vi "ADCP过程数据.vi"(7 "电压":sgl, 8 "Error in":errorcluster caption="Error in (no error)", 9 "纵摇":sgl, 10 "横摇":sgl, 11 "时间":timestamp) -> (0 "错误输出":errorcluster)   [LabVIEW 2016, in "ADCP.lvlib"]
uses:
  ADCP.lvlib
panel:
  out "data":T1
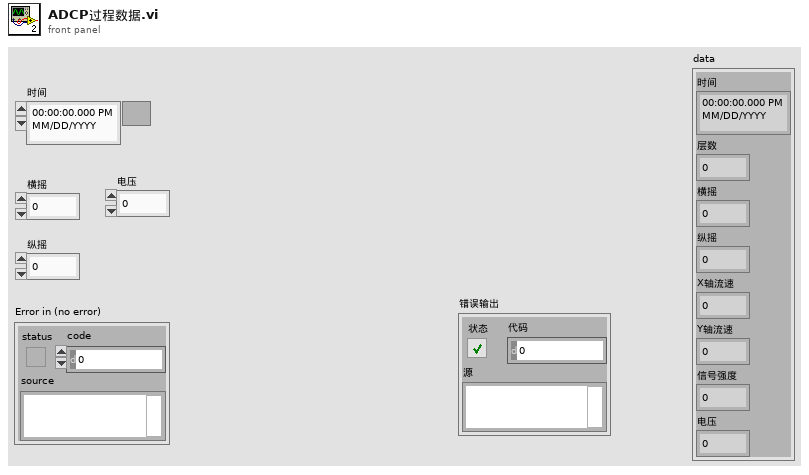
[diagram p1: front panel]
types:
  T1 = cluster{"时间":timestamp, "层数":u16, "横摇":sgl, "纵摇":sgl, "X轴流速":sgl, "Y轴流速":sgl, "信号强度":u16, "电压":sgl}
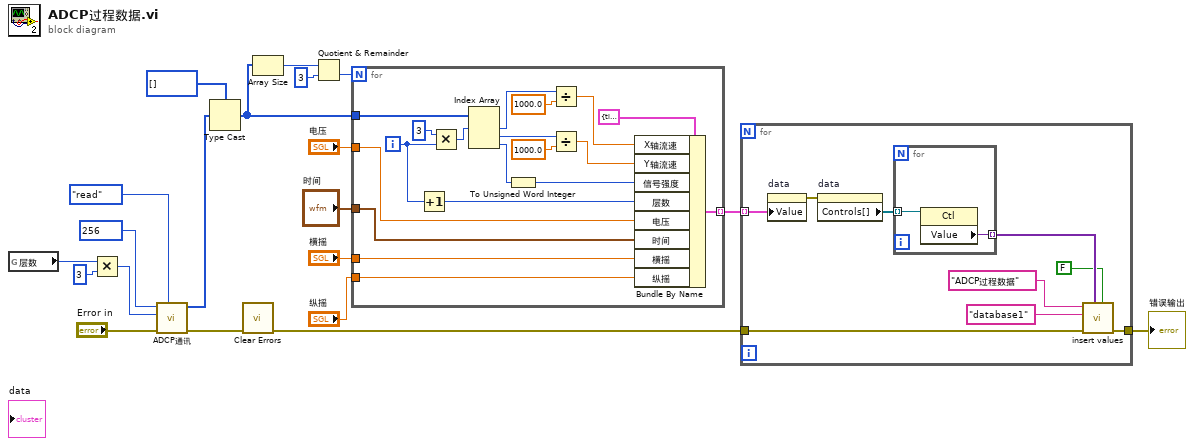
[diagram p0: block diagram]
diagram:
  n1 = global read "ADCP全局变量.vi" "层数"() -> (w19:u16)
  n2 = Multiply(x=w19, y=u16 3) -> (x*y=w17:u16)
  n3 = call "ADCP通讯.vi"("STEP"=enum16{"open", "read", "write", "close"}."read", "Error in"="Error in", "quantity"=w17, "starting address"=u16 256) -> ("error out"=w2:errorcluster, "Registers"=w10:u16[])  [unwired: 5 in, 1 out]
  n4 = Type Cast(type=i16[] [], x=w10) -> (*(type *) &x=w14:i16[])
  n5 = call <vilib>:"Clear Errors.vi"("error in (no error)"=w2) -> ("error out"=w1:errorcluster)  [unwired: 5 in, 1 out]
  n6 = Array Size(array=w14) -> (size(s)=w13:i32)
  n7 = Quotient & Remainder(x=w13, y=3) -> (floor(x/y)=w11:i32)  [unwired: 1 out]
  n8 = for {
    N: w11 -> [_]
    tunnel: w14 -> [w39]
    tunnel: [w27] -> w6 mode=indexing
    tunnel: "电压" -> [w26]
    tunnel: "时间" -> [w25]
    tunnel: "横摇" -> [w24]
    tunnel: "纵摇" -> [w23]
    i -> [w22]
    n9 = Increment(x=w22) -> (x+1=w21:i32)
    n10 = Multiply(x=3, y=w22) -> (x*y=w37:i32)
    n11 = Index Array(array=w39, index #1=w37) -> (element #1=w36:i16, element #2=w33:i16, element #3=w32:i16)  [unwired: 2 in]
    n12 = To Unsigned Word Integer(number=w32) -> (unsigned 16bit integer=w28:u16)
    n13 = Divide(x=w36, y=sgl 1000.0) -> (x/y=w30:sgl)
    n14 = Divide(x=w33, y=sgl 1000.0) -> (x/y=w29:sgl)
    n15 = Bundle By Name(cluster=T1 {"时间"=timestamp(0 s since 1904-01-01), "层数"=0, "横摇"=0.0, "纵摇"=0.0, "X轴流速"=0.0, "Y轴流速"=0.0, "信号强度"=0, "电压"=0.0}, "X轴流速"=w30, "Y轴流速"=w29, "信号强度"=w28, "层数"=w21, "电压"=w26, "时间"=w25, "横摇"=w24, "纵摇"=w23) -> (w27:T1)
  }
  n16 = for {
    tunnel: w6 -> [w46] mode=indexing
    tunnel: w1 -> [w41]
    tunnel: [w40] -> w4
    n17 = property on="data" class="Clust (严格)"("Value"=w46) -> (error out=w45:errorcluster)  [unwired: 2 in, 1 out]
    n18 = property on="data" class="Clust (严格)"(error in=w45) -> ("Controls[]"=w44:refnum<vi>[])  [unwired: 1 in, 2 out]
    n19 = for {
      tunnel: w44 -> [w50] mode=indexing
      tunnel: [w49] -> w43 mode=indexing
      n20 = property class="Ctl"(reference=w50) -> ("Value"=w49:variant)  [unwired: 1 in, 2 out]
    }
    n21 = call "insert values.vi"("是否创建唯一键"=FALSE, "data"=w43, "错误输入（无错误）"=w41, "database"="database1", "Tabe Name"="ADCP过程数据") -> ("错误输出"=w40:errorcluster)  [unwired: 6 in]
  }
  "错误输出" <- w4
